vi "WriteIQ_sglwfm.vi"(8 "error in (no error)":errorcluster, 10 "IQ wfm":waveform(csg), 11 "reference in":refnum<class "IQBurst_memo.lvclass">) -> (0 "error out":errorcluster, 3 "reference out":refnum<class "IQBurst_memo.lvclass">)   [LabVIEW 2019, in "IQBurst_memo.lvclass"]
doc: "Writes IQ data to object"
uses:
  IQBurst_memo.lvclass
  C:/Barkhausen mmWave radar/Development/LV/Barkhausen mmWave hardware control/Host/SubVIs/mmWave data_class/mmWave data.lvclass
  mmWave data_class/mmWave data.lvclass
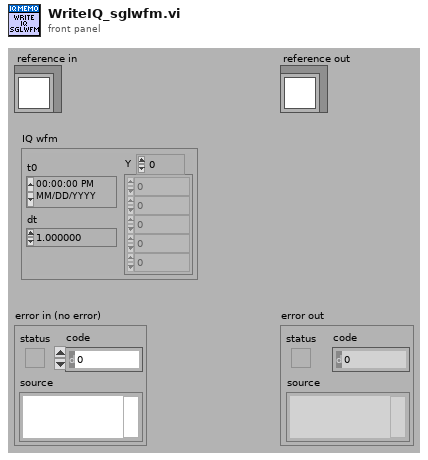
[diagram p1: front panel]
types:
  T1 = typedef "mmWave data.lvclass/ObjectAttributesRef.ctl" = refnum<data-value>
  T2 = typedef "IQBurst_memo.lvclass/ObjectAttributesRef.ctl" = refnum<data-value>
  T3 = typedef "IQBurst_memo.lvclass/ObjectAttributes.ctl" = cluster{"IQ data":i16[], "dt":dbl}
  T4 = typedef "mmWave data.lvclass/ObjectAttributes.ctl" = cluster{"MyAttribute":dbl, "size":i32}
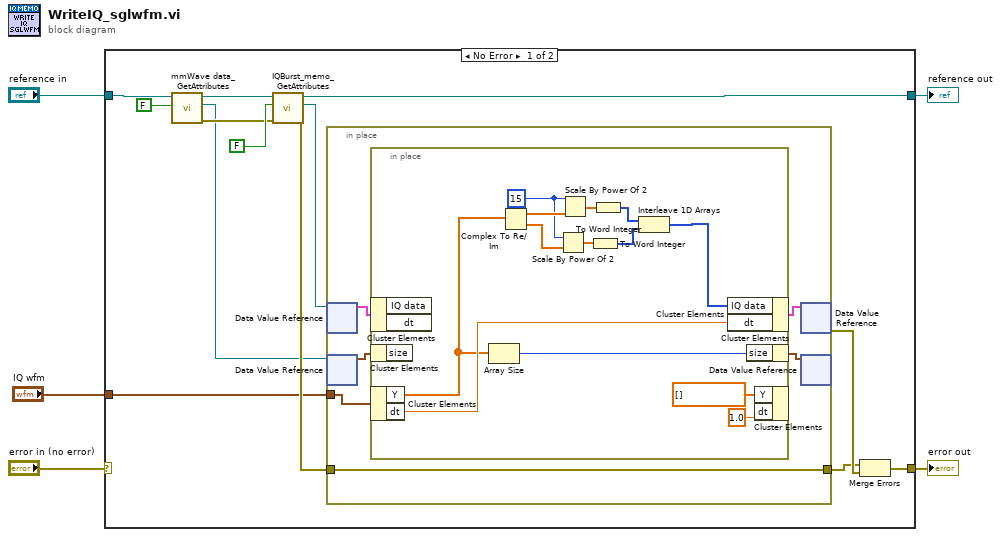
[diagram p0: block diagram]
diagram:
  n1 = case shown="No Error" "error in (no error)" {
    selector: "error in (no error)" -> [_ w39]
    tunnel: [w18 w39] -> w4
    tunnel: [w12 w38] -> w2
    tunnel: "reference in" -> [w15 w38]
    tunnel: "IQ wfm" -> [w6 _]
    frame No Error {
      n2 = call "mmWave data_GetAttributes.vi"("return data? (T)"=FALSE, "reference in"=w15) -> ("error out"=w8:errorcluster, "attributes ref"=w7:T1, "reference out"=w10:refnum<class "IQBurst_memo.lvclass">)  [unwired: 6 in, 1 out]
      n3 = call "IQBurst_memo_GetAttributes.vi"("error in (no error)"=w8, "return data? (T)"=FALSE, "reference in"=w10) -> ("error out"=w13:errorcluster, "attributes ref"=w11:T2, "reference out"=w12:refnum<class "IQBurst_memo.lvclass">)  [unwired: 5 in, 1 out]
      n4 = in-place {
        in-place-border: w13 -> [w22]
        in-place-border: [w22] -> w16
        in-place-border: w6 -> [w20]
        n5 = in-place-dvr #1(w11) -> (w23:T3)  [unwired: 1 out]
        n6 = in-place-dvr #2(w7) -> (w21:T4)  [unwired: 1 out]
        n7 = in-place {
          w29 = i16 15 ("n")
          n8 = in-place-cluster #3(w23) -> ()  [unwired: 2 out]
          n9 = in-place-cluster #4(w21) -> ()  [unwired: 1 out]
          n10 = in-place-cluster #5(w20) -> ("Y"=w33:csg[], "dt"=w37:dbl)
          n11 = Array Size(array=w33) -> (size(s)=w34:i32)
          n12 = Complex To Re/Im(x + iy=w33) -> (x=w31:sgl[], y=w30:sgl[])
          n13 = Scale By Power Of 2(n=w29, x=w30) -> (x*2^n=w27:sgl[])
          n14 = Scale By Power Of 2(n=w29, x=w31) -> (x*2^n=w28:sgl[])
          n15 = To Word Integer(number=w27) -> (16bit integer=w25:i16[])
          n16 = To Word Integer(number=w28) -> (16bit integer=w26:i16[])
          n17 = Interleave 1D Arrays(w26, w25) -> (w32:i16[])
          n18 = in-place-cluster #3("IQ data"=w32, "dt"=w37) -> (w24:T3)
          n19 = in-place-cluster #4("size"=w34) -> (w19:T4)
          n20 = in-place-cluster #5("Y"=csg[] [], "dt"=1.0) -> ()  [unwired: 1 out]
        }
        n21 = in-place-dvr #1(w24) -> (w17:errorcluster)  [unwired: 1 out]
        n22 = in-place-dvr #2(w19) -> ()  [unwired: 2 out]
      }
      n23 = Merge Errors(w16, w17) -> (w18:errorcluster)
    }
    frame Error {
    }
  }
  "error out" <- w4
  "reference out" <- w2
